vi "GetCellStrColor.vi"(7 "Color":u32, 8 "error in (no error)":errorcluster, 10 "Hdr Name":T1, 11 "Channel in":refnum<class "Channel.lvclass">) -> (0 "error out":errorcluster, 1 "Cell String":string, 2 "Cell Color":u32, 3 "Channel out":refnum<class "Channel.lvclass">)   [LabVIEW 2012, in "Measurement Channels.lvlib" / "Channel.lvclass"]
uses:
  Channel.lvclass
  Common/Controls/HeaderNames.ctl
  Channel.lvclass/Channel.ctl
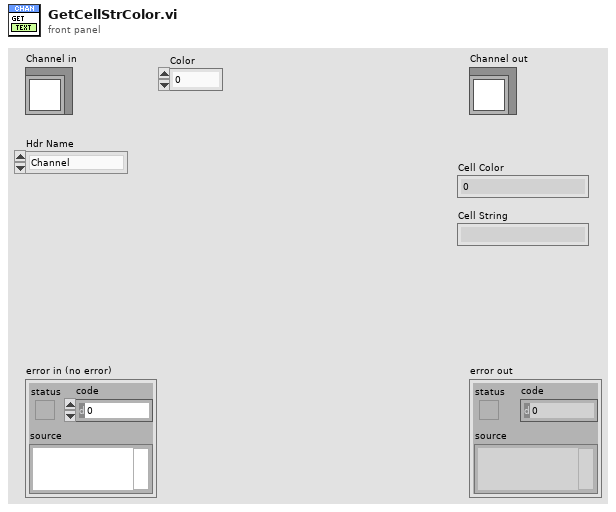
[diagram p1: front panel]
types:
  T1 = typedef "HeaderNames.ctl" = enum16{"Channel", "Device", "Spacer", "Description", "MB", "Range", "Terminal", "Coupling", "Thresh (V)", "Pulse/Rev", "Slope", "Min EU", "Min RPM", "mV/EU", "Iex", "Temp Units", "Type", "CJC Src", "CJC Val", "Ro", "Wire Cfg", "Strain Mode", "Vex", "Bridge Type", "GF", "Gauge Res", "Poisson", "Lead Res", "Init Strain", "GAF", "Scale", "Offset", "Unit (EU)", "dB?", "dB Ref", "Cal Mag", "Cal Units", "Max Temp", "Min Temp", "Max Strain", "Min Strain"}
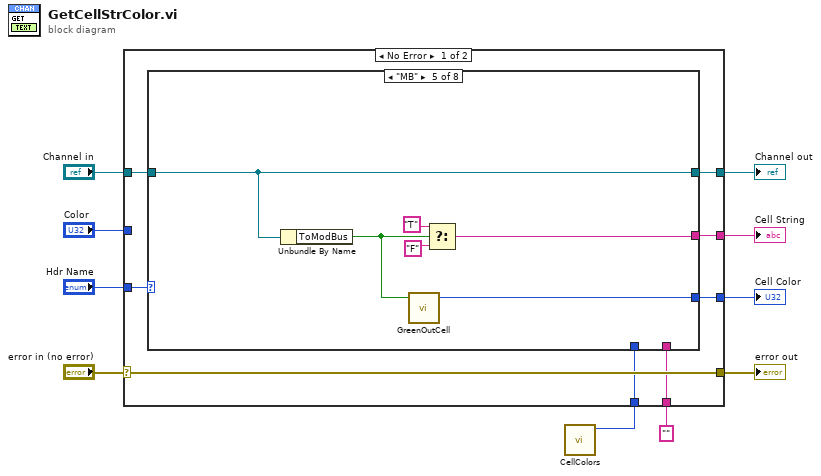
[diagram p0: block diagram]
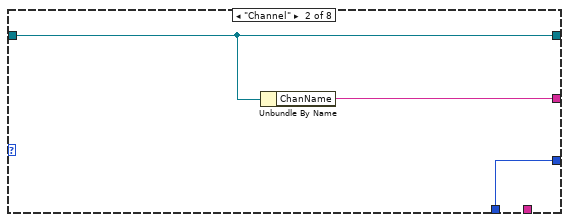
[diagram p3: hidden frame]
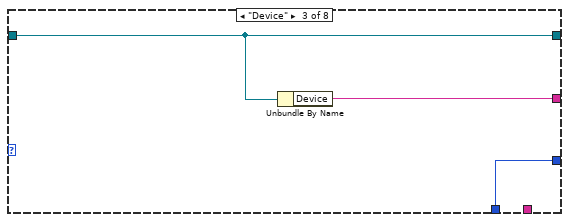
[diagram p4: hidden frame]
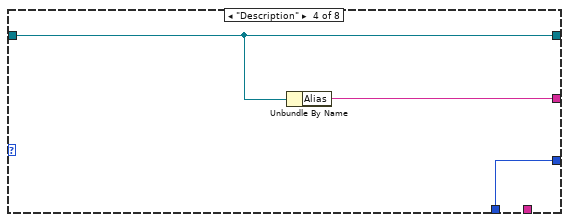
[diagram p5: hidden frame]
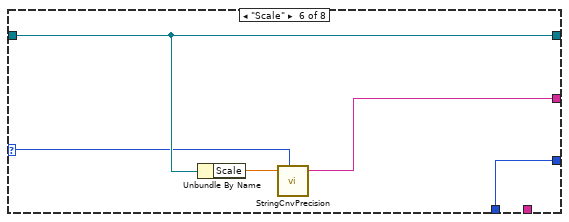
[diagram p6: hidden frame]
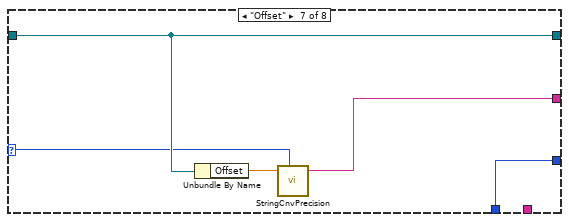
[diagram p7: hidden frame]
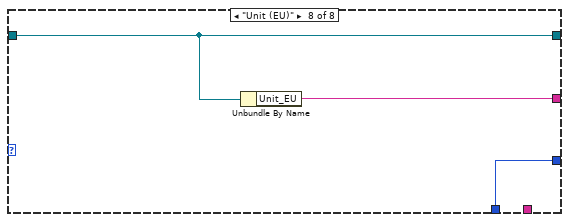
[diagram p8: hidden frame]
diagram:
  n1 = call "CellColors.vi"() -> ("Normal"=w3:u32)  [unwired: 8 in, 3 out]
  n2 = case shown="No Error" "error in (no error)" {
    selector: "error in (no error)" -> [w18 w53]
    tunnel: [w18 w53] -> w9
    tunnel: [w16 w52] -> w7
    tunnel: "Channel in" -> [w17 w52]
    tunnel: "Hdr Name" -> [w15 _]
    tunnel: [w14 w51] -> w5
    tunnel: [w13 w50] -> w4
    tunnel: w3 -> [w12 w50]
    tunnel: "" ("Alias") -> [w11 w51]
    tunnel: "Color" -> [_ _]
    frame No Error {
      n3 = case shown="\"MB\"" w15 {
        selector: w15 -> [_ _ _ _ _ w39 w44 _]
        tunnel: w17 -> [w21 w24 w27 w30 w36 w41 w46 w48]
        tunnel: [w21 w24 w27 w30 w36 w41 w46 w48] -> w16
        tunnel: [w20 w23 w26 w29 w33 w38 w43 w47] -> w14
        tunnel: [w19 w22 w25 w28 w31 w37 w42 w49] -> w13
        tunnel: w12 -> [w19 w22 w25 w28 _ w37 w42 w49]
        tunnel: w11 -> [w20 _ _ _ _ _ _ _]
        frame Default {
        }
        frame "Channel" {
          n4 = Unbundle By Name(w24) -> ("ChanName"=w23:string)
        }
        frame "Device" {
          n5 = Unbundle By Name(w27) -> ("Device"=w26:string)
        }
        frame "Description" {
          n6 = Unbundle By Name(w30) -> ("Alias"=w29:string)
        }
        frame "MB" {
          n7 = Unbundle By Name(w36) -> ("ToModBus"=w32:bool)
          n8 = call "GreenOutCell.vi"("ToModBus?"=w32) -> ("Color"=w31:u32)  [unwired: 4 in]
          n9 = Select(t="T", s=w32, f="F") -> (s? t:f=w33:string)
        }
        frame "Scale" {
          n10 = Unbundle By Name(w41) -> ("Scale"=w40:dbl)
          n11 = call "StringCnvPrecision.vi"("Number"=w40, "Header"=w39) -> ("Float String"=w38:string)  [unwired: 5 in]
        }
        frame "Offset" {
          n12 = Unbundle By Name(w46) -> ("Offset"=w45:dbl)
          n13 = call "StringCnvPrecision.vi"("Number"=w45, "Header"=w44) -> ("Float String"=w43:string)  [unwired: 5 in]
        }
        frame "Unit (EU)" {
          n14 = Unbundle By Name(w48) -> ("Unit_EU"=w47:string)
        }
      }
    }
    frame Error {
    }
  }
  "error out" <- w9
  "Channel out" <- w7
  "Cell String" <- w5
  "Cell Color" <- w4
